vi "Cache_PPL Global_List Cache Files.vi"(8 "error in (no error)":errorcluster) -> (0 "error out":errorcluster, 3 "Cache Paths":path[](array[path]))   [LabVIEW 2019, in "ClassLoader.lvlib"]
doc: "Return paths to the ini cache files for all loaded PPLs."
uses:
  ClassLoader.lvlib
  Cache_PPL Global.vi
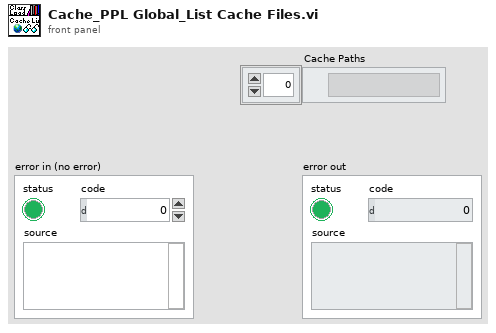
[diagram p1: front panel]
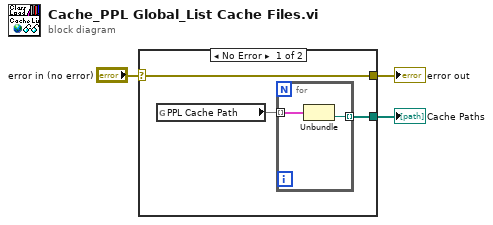
[diagram p0: block diagram]
diagram:
  n1 = case shown="No Error" "error in (no error)" {
    selector: "error in (no error)" -> [w5 w9]
    tunnel: [w5 w9] -> w2
    tunnel: [w4 _] -> w1
    frame No Error {
      n2 = global read "Cache_PPL Global.vi" "PPL Cache Path"() -> (w6:map{string, path})
      n3 = for {
        tunnel: w6 -> [w8] mode=indexing
        tunnel: [w7] -> w4 mode=indexing
        n4 = Unbundle(w8) -> ("value"=w7:path)  [unwired: 1 out]
      }
    }
    frame Error {
    }
  }
  "error out" <- w2
  "Cache Paths" <- w1
